vi "Get Memory Size of Variant.vi"(8 "error in (no error)":errorcluster, 11 "data":variant) -> (0 "error out":errorcluster, 1 "byte_alignment":i16, 2 "flatten_string_size":i32, 3 "mem_size":i64)   [LabVIEW 2021, in "DataTypes_CIF_U.lvlib"]
doc: "Same functionality as Fixed Size Sizeof.vim, however now a variant input is used and dependency on malleable VIs are avoided."
uses:
  DataTypes_CIF_U.lvlib
  Typedef/Errors.ctl
  Errors/Append Error Location.vi
  <vilib>/Utility/Data Type/NI_Data Type.lvlib
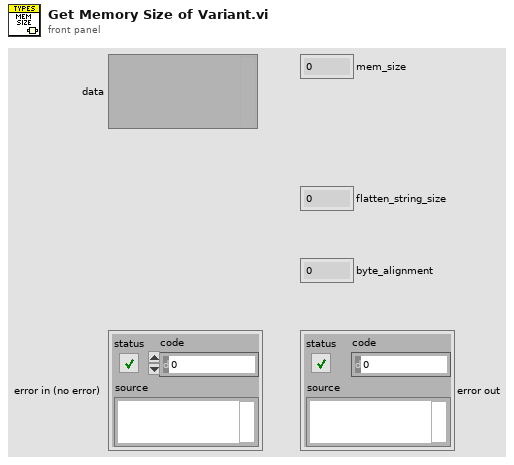
[diagram p1: front panel]
types:
  T1 = typedef "NI_Data Type.lvlib/Data Type.ctl" = enum8{"Invalid Type", "Void", "I8", "I16", "I32", "I64", "U8", "U16", "U32", "U64", "Single Float", "Double Float", "Extended Float", "Single Complex", "Double Complex", "Extended Complex", "Enum U8", "Enum U16", "Enum U32", "Enum U64", "Single Float With Unit", "Double Float With Unit", "Extended Float With Unit", "Single Complex with Unit", "Double Complex with Unit", "Extended Complex with Unit", "Boolean", "String", "Path", "Picture", "Tag", "Array", "Cluster", "Variant", "LV Variant", "Waveform", "Timestamp", "Digital Waveform", "Digital Data", "ExpressData", "Refnum", "External Data", "VI", "Poly VI", "LabVIEW Class Instance", "Fixed Point", "Set Collection", "Map Collection"}
  T2 = typedef "DataTypes_CIF_U.lvlib/Errors.ctl" = enum16{"Too few bytes", "Unsupported Type"}
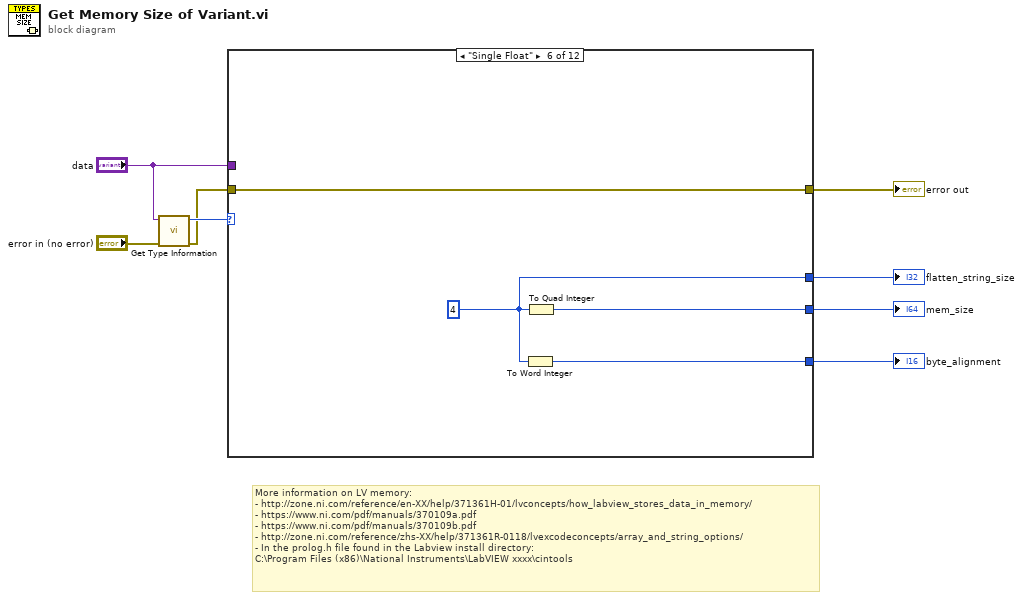
[diagram p0: block diagram]
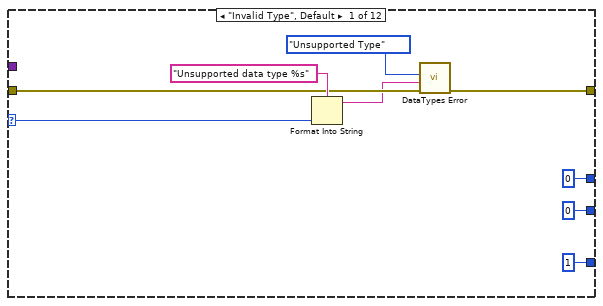
[diagram p2: hidden frame]
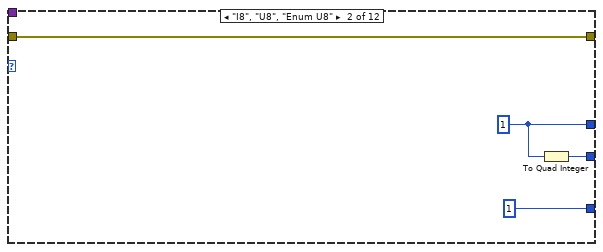
[diagram p3: hidden frame]
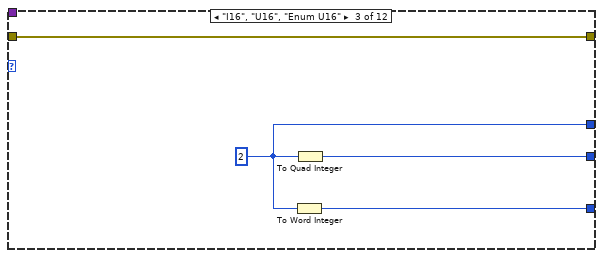
[diagram p4: hidden frame]
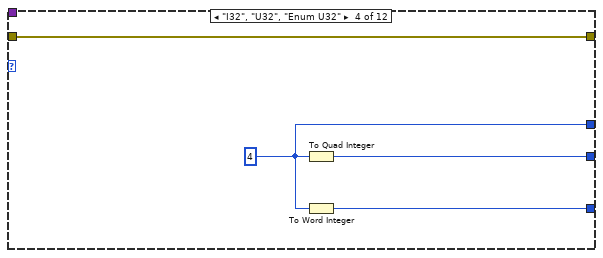
[diagram p5: hidden frame]
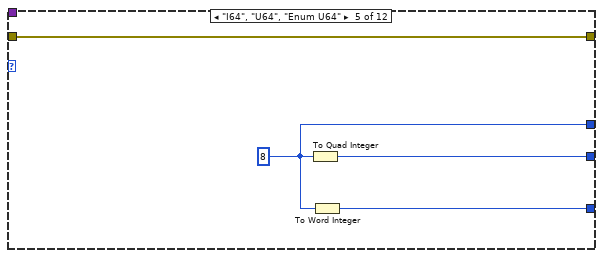
[diagram p6: hidden frame]
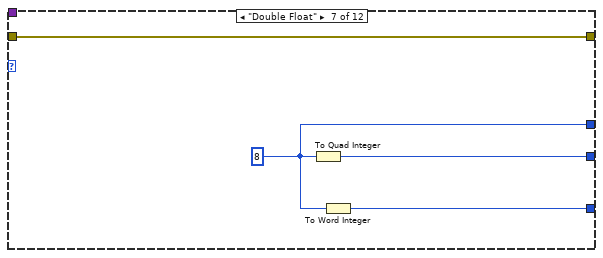
[diagram p7: hidden frame]
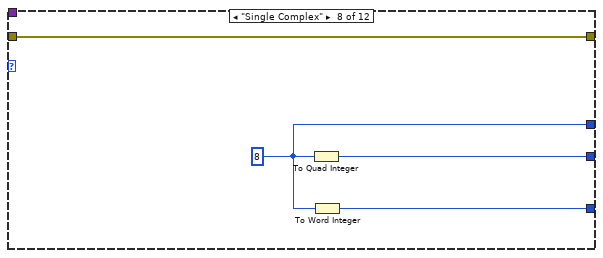
[diagram p8: hidden frame]
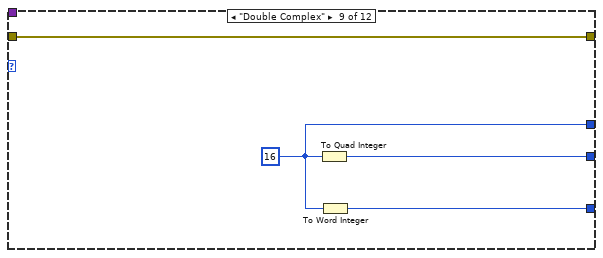
[diagram p9: hidden frame]
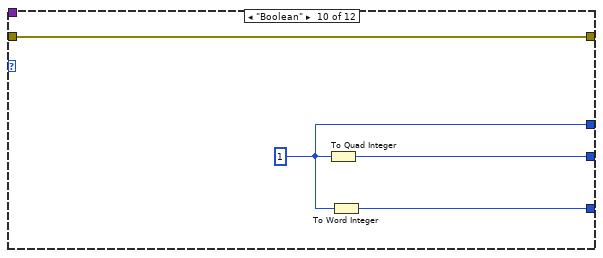
[diagram p10: hidden frame]
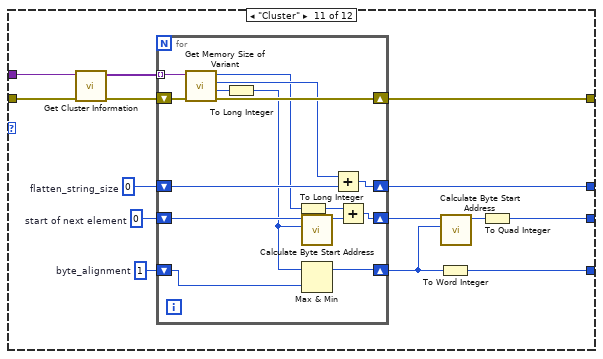
[diagram p11: hidden frame]
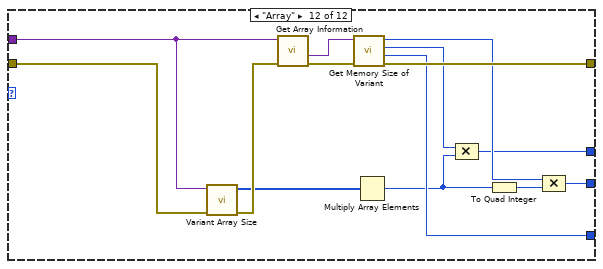
[diagram p12: hidden frame]
diagram:
  # "More information on LV memory:\n- http://zone.ni.com/reference/en-XX/help/371361H-01/lvconcepts/how_labview_stores_data_in_memory/\n- https://www.ni.com/pdf/manuals/370109a.pdf \n- https://www.ni.com/pdf/manuals/370109b.pdf\n- http://zone.ni.com/reference/zhs-XX/help/371361R-0118/lvexcodeconcepts/array_and_string_options/\n- In the prolog.h file found in the Labview install directory:\nC:\\Program Files (x86)\\National Instruments\\LabVIEW xxxx\\cintools"
  n1 = call <vilib>:"Get Type Information.vi"("error in (no error)"="error in (no error)", "variant"="data") -> ("error out"=w1:errorcluster, "type"=w8:T1)  [unwired: 5 in, 3 out]
  n2 = case shown="\"Single Float\"" w8 {
    selector: w8 -> [w16 _ _ _ _ _ _ _ _ _ _ _]
    tunnel: w1 -> [w11 w20 w25 w29 w33 w37 w41 w45 w49 w53 w64 w87]
    tunnel: [w10 w20 w25 w29 w33 w37 w41 w45 w49 w53 w65 w94] -> w7
    tunnel: [0 ("flatten_string_size") w21 w24 w28 w32 w36 w40 w44 w48 w52 w60 w90] -> w6
    tunnel: [i64 0 ("flatten_string_size") w18 w22 w26 w30 w35 w38 w43 w47 w50 w54 w92] -> w5
    tunnel: [i16 1 ("flatten_string_size") i16 1 ("flatten_string_size") w23 w27 w31 w34 w39 w42 w46 w51 w55 w93] -> w4
    tunnel: "data" -> [_ _ _ _ _ _ _ _ _ _ w67 w88]
    frame "Invalid Type", Default {
      n3 = Format Into String(format string="Unsupported data type %s", w16) -> (resulting string=w9:string)  [unwired: 2 in, 1 out]
      n4 = call "DataTypes Error.vi"("error in (no error)"=w11, "String to Append"=w9, "Error"=Errors."Unsupported Type") -> ("error out"=w10:errorcluster)  [unwired: 8 in]
    }
    frame "I8", "U8", "Enum U8" {
      w21 = 1 ("flatten_string_size")
      n5 = To Quad Integer(1:w21) -> (0:w18:i64)
    }
    frame "I16", "U16", "Enum U16" {
      w24 = 2 ("flatten_string_size")
      n6 = To Word Integer(number=w24) -> (16bit integer=w23:i16)
      n7 = To Quad Integer(1:w24) -> (0:w22:i64)
    }
    frame "I32", "U32", "Enum U32" {
      w28 = 4 ("flatten_string_size")
      n8 = To Quad Integer(1:w28) -> (0:w26:i64)
      n9 = To Word Integer(number=w28) -> (16bit integer=w27:i16)
    }
    frame "I64", "U64", "Enum U64" {
      w32 = 8 ("flatten_string_size")
      n10 = To Quad Integer(1:w32) -> (0:w30:i64)
      n11 = To Word Integer(number=w32) -> (16bit integer=w31:i16)
    }
    frame "Single Float" {
      w36 = 4 ("flatten_string_size")
      n12 = To Word Integer(number=w36) -> (16bit integer=w34:i16)
      n13 = To Quad Integer(1:w36) -> (0:w35:i64)
    }
    frame "Double Float" {
      w40 = 8 ("flatten_string_size")
      n14 = To Quad Integer(1:w40) -> (0:w38:i64)
      n15 = To Word Integer(number=w40) -> (16bit integer=w39:i16)
    }
    frame "Single Complex" {
      w44 = 8 ("flatten_string_size")
      n16 = To Quad Integer(1:w44) -> (0:w43:i64)
      n17 = To Word Integer(number=w44) -> (16bit integer=w42:i16)
    }
    frame "Double Complex" {
      w48 = 16 ("flatten_string_size")
      n18 = To Quad Integer(1:w48) -> (0:w47:i64)
      n19 = To Word Integer(number=w48) -> (16bit integer=w46:i16)
    }
    frame "Boolean" {
      w52 = 1 ("flatten_string_size")
      n20 = To Quad Integer(1:w52) -> (0:w50:i64)
      n21 = To Word Integer(number=w52) -> (16bit integer=w51:i16)
    }
    frame "Cluster" {
      w59 = 1  # byte_alignment
      w61 = 0  # flatten_string_size
      w62 = 0  # start of next element
      n22 = call <vilib>:"Get Cluster Information.vi"("error in (no error)"=w64, "variant"=w67) -> ("error out"=w63:errorcluster, "cluster elements"=w66:variant[])  [unwired: 8 in]
      n23 = for {
        tunnel: w66 -> [w82] mode=indexing
        shift-right: [w80] -> w65
        shift-left: w63 -> [w81]
        shift-right: [w73] -> w58
        shift-left: w62 -> [w72]
        shift-right: [w78] -> w60
        shift-left: w61 -> [w79]
        shift-right: [w75] -> w57
        shift-left: w59 -> [w76]
        n24 = call "Get Memory Size of Variant.vi"("error in (no error)"=w81, "data"=w82) -> ("error out"=w80:errorcluster, "byte_alignment"=w71:i16, "flatten_string_size"=w77:i32, "mem_size"=w74:i64)  [unwired: 6 in]
        n25 = To Long Integer(number=w71) -> (32bit integer=w68:i32)
        n26 = To Long Integer(number=w74) -> (32bit integer=w69:i32)
        n27 = call "Calculate Byte Start Address.vi"("data_byte_alignment"=w68, "byte_address_start"=w72) -> ("byte_address_data"=w70:i32)  [unwired: 7 in, 1 out]
        n28 = Max & Min(x=w68, y=w76) -> (max(x,y)=w75:i32)  [unwired: 1 out]
        n29 = Add(x=w77, y=w79) -> (x+y=w78:i32)
        n30 = Add(x=w69, y=w70) -> (x+y=w73:i32)
      }
      n31 = To Word Integer(number=w57) -> (16bit integer=w55:i16)
      n32 = call "Calculate Byte Start Address.vi"("data_byte_alignment"=w57, "byte_address_start"=w58) -> ("byte_address_data"=w56:i32)  [unwired: 7 in, 1 out]
      n33 = To Quad Integer(1:w56) -> (0:w54:i64)
    }
    frame "Array" {
      n34 = call "Variant Array Size.vi"("error in (no error)"=w87, "data"=w88) -> ("error out"=w86:errorcluster, "lengths"=w84:i32[])  [unwired: 7 in, 1 out]
      n35 = call <vilib>:"Get Array Information.vi"("error in (no error)"=w86, "variant"=w88) -> ("error out"=w95:errorcluster, "array element data type"=w96:variant)  [unwired: 6 in, 2 out]
      n36 = call "Get Memory Size of Variant.vi"("error in (no error)"=w95, "data"=w96) -> ("error out"=w94:errorcluster, "byte_alignment"=w93:i16, "flatten_string_size"=w89:i32, "mem_size"=w91:i64)  [unwired: 6 in]
      n37 = Multiply Array Elements(1:w84) -> (0:w83:i32)
      n38 = Compound Arithmetic op=MULTIPLY(w89, w83) -> (w90:i32)
      n39 = To Quad Integer(1:w83) -> (0:w85:i64)
      n40 = Compound Arithmetic op=MULTIPLY(w91, w85) -> (w92:i64)
    }
  }
  "error out" <- w7
  "flatten_string_size" <- w6
  "mem_size" <- w5
  "byte_alignment" <- w4
